vi "Get.vi"(8 "error in (no error)":errorcluster, 11 "Template":refnum<class "Singleton.lvclass">) -> (0 "error out":errorcluster, 3 "object":refnum<class "Singleton.lvclass">)   [LabVIEW 2014, in "Singleton.lvlib" / "Singleton.lvclass"]
uses:
  Singleton.lvclass
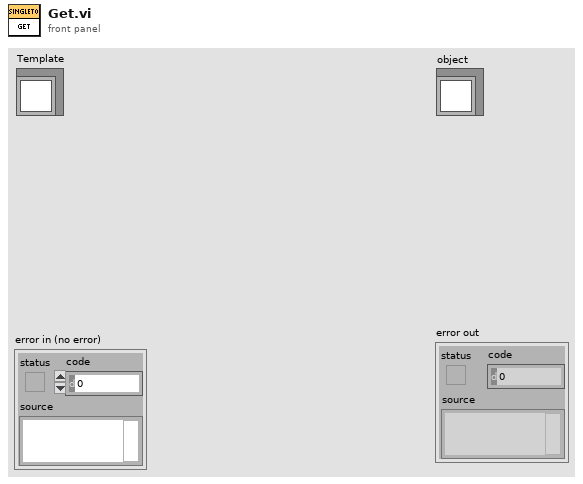
[diagram p1: front panel]
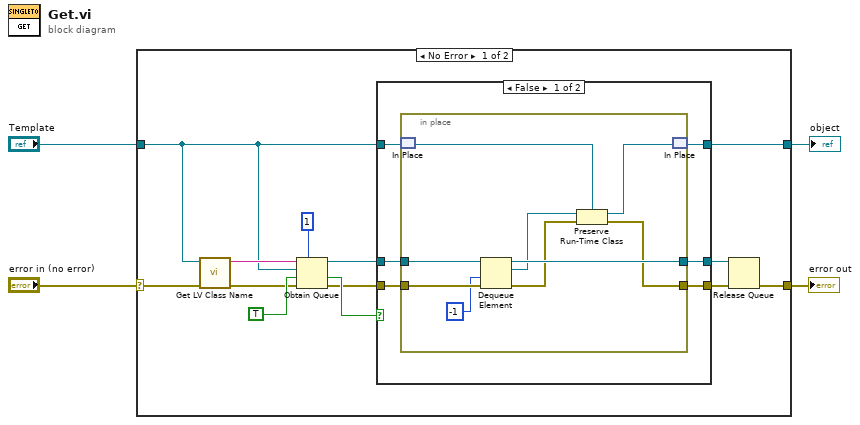
[diagram p0: block diagram]
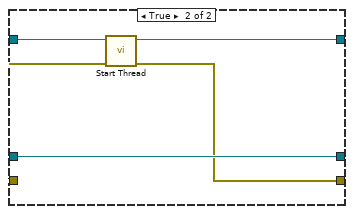
[diagram p2: hidden frame]
diagram:
  n1 = case shown="No Error" "error in (no error)" {
    selector: "error in (no error)" -> [w14 w39]
    tunnel: [w5 w39] -> w3
    tunnel: "Template" -> [w6 w38]
    tunnel: [w7 w38] -> w1
    frame No Error {
      n2 = call <vilib>:"Get LV Class Name.vi"("error in (no error)"=w14, "object"=w6) -> ("error out"=w13:errorcluster, "class name"=w17:string)  [unwired: 8 in]
      n3 = Obtain Queue(max queue size (-1, unlimited)=1, name (unnamed)=w17, element data type=w6, create if not found? (T)=TRUE, error in (no error)=w13) -> (queue out=w10:refnum<queue>, created new?=w12:bool, error out=w11:errorcluster)
      n4 = case shown="False" w12 {
        tunnel: w11 -> [w22 w34]
        tunnel: w10 -> [w23 w37]
        tunnel: [w18 w36] -> w7
        tunnel: [w21 w35] -> w9
        tunnel: w6 -> [w19 w33]
        tunnel: [w20 w37] -> w8
        frame False {
          n5 = in-place {
            in-place-border: w23 -> [w32]
            in-place-border: w22 -> [w31]
            in-place-border: [w24] -> w21
            in-place-border: [w30] -> w20
            n6 = in-place-match #1(w19) -> (w28:refnum<class "Singleton.lvclass">)
            n7 = Dequeue Element(queue=w32, timeout in ms (-1)=-1, error in (no error)=w31) -> (queue out=w30:refnum<queue>, element=w27:refnum<class "Singleton.lvclass">, error out=w25:errorcluster)  [unwired: 1 out]
            n8 = Preserve Run-Time Class(object in=w27, error in=w25, 2:w28) -> (object out=w26:refnum<class "Singleton.lvclass">, error out=w24:errorcluster)
            n9 = in-place-match #1(w26) -> (w18:refnum<class "Singleton.lvclass">)
          }
        }
        frame True {
          n10 = call "Start Thread.vi"("error in (no error)"=w34, "Template"=w33) -> ("error out"=w35:errorcluster, "object"=w36:refnum<class "Singleton.lvclass">)  [unwired: 8 in]
        }
      }
      n11 = Release Queue(queue=w8, error in (no error)=w9) -> (error out=w5:errorcluster)  [unwired: 1 in, 2 out]
    }
    frame Error {
    }
  }
  "error out" <- w3
  "object" <- w1
